vi "string_signal.vi"(5 "Offset":dbl, 7 "Phase":dbl, 8 "Error In":errorcluster, 9 "Waveform":T1(ring), 10 "Hz String":string, 11 "Amp String":string) -> (0 "Error Out":errorcluster, 3 "Signal String":string)   [LabVIEW 2021, in "Signal.lvlib"]
doc: "This subVI is used for forming the signal properties string."
uses:
  Signal.lvlib
panel:
  # "Input"
  # "Output"
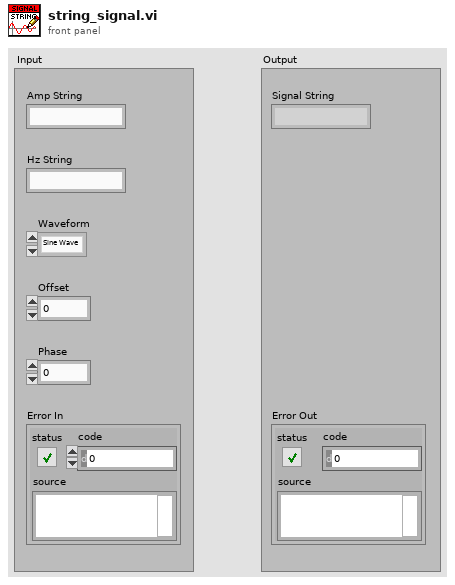
[diagram p1: front panel]
types:
  T1 = enum16{"Sine Wave", "Triangle Wave", "Square Wave", "Sawtooth Wave"}
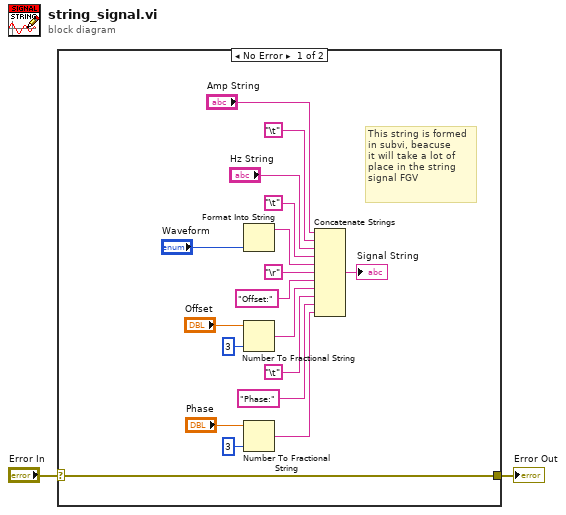
[diagram p0: block diagram]
diagram:
  n1 = case shown="No Error" "Error In" {
    selector: "Error In" -> [w11 w21]
    tunnel: [w11 w21] -> w1
    frame No Error {
      # "This string is formed\nin subvi, beacuse\nit will take a lot of\nplace in the string \nsignal FGV"
      n2 = Format Into String("Waveform") -> (resulting string=w5:string)  [unwired: 3 in, 1 out]
      n3 = Number To Fractional String(number="Offset", precision (6)=i16 3) -> (F-format string=w16:string)  [unwired: 2 in]
      n4 = Number To Fractional String(number="Phase", precision (6)=i16 3) -> (F-format string=w20:string)  [unwired: 2 in]
      n5 = Concatenate Strings("Amp String", "\t", "Hz String", "\t", w5, "\r", "Offset:", w16, "\t", "Phase:", w20) -> (→"Signal String":string)
    }
    frame Error {
    }
  }
  "Error Out" <- w1
